vi "FromRepo.vi"(8 "error in":errorcluster, 9 "from repo cluster":T2, 10 "repository in":refnum<class "CEF_Repository.lvclass">, 11 "CEF_configuration":refnum<class "CEF_serializable node.lvclass">) -> (0 "error out":errorcluster, 2 "repository out":refnum<class "CEF_Repository.lvclass">, 3 "node":T1)   [LabVIEW 2023, in "CEF.lvlib" / "CEF_serializable node.lvclass"]
doc: "Grabs information from the Repo and stores it in the nodes.Copyright 2017 National Instruments Corporation\n\nLicensed under the Apache License, Version 2.0 (the \"License\"); you may not use this file except in compliance with the License. You may obtain a copy of the License at http://www.apache.org/licenses/LICENSE-2.0\nUnless required by applicable law or agreed to in writing, software distributed under the License is distributed on an \"AS IS\" BASIS, WITHOUT WARRANTIES OR CONDITIONS OF ANY KIND, either express or implied. See the License for the specific language governing permissions and limitations under the License."
uses:
  CEF_serializable node.lvclass
  Repository/CEF_Repository.lvclass
  Node/FromRepoCluster.ctl
  Node/NodeRef.ctl
  Node/CEF_Node.lvclass
  hierarchy repo/CEF_HierarchyRepo.lvclass
  C:/Working Copy/TSS/Utilities/Configuration Framework/Repository/CEF_Repository.lvclass
  serializable configuration/CEF_serializable configuration.lvclass
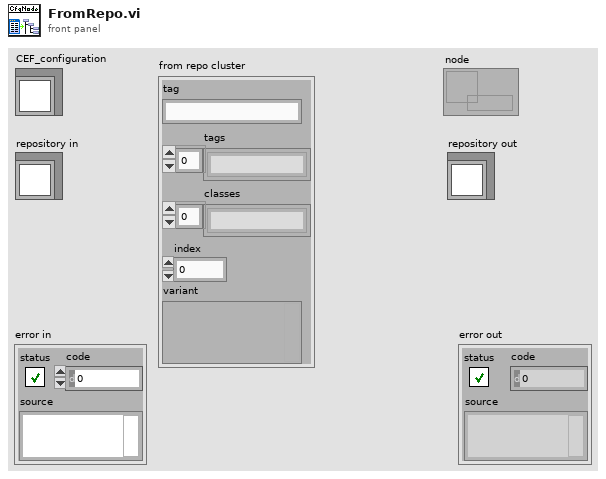
[diagram p1: front panel]
types:
  T1 = typedef "CEF.lvlib/CEF_Node.lvclass/NodeRef.ctl" = refnum<data-value>
  T2 = typedef "CEF.lvlib/CEF_Node.lvclass/FromRepoCluster.ctl" = cluster{"tag":string, "tags":string[], "classes":string[], "index":i32, "variant":variant}
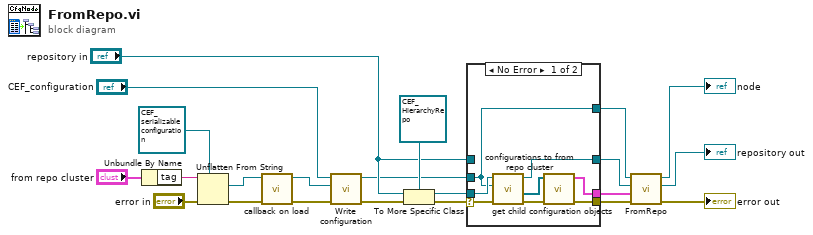
[diagram p0: block diagram]
diagram:
  n1 = Unbundle By Name("from repo cluster") -> ("tag"=w9:string)
  n2 = Unflatten From String(type=refnum<class "CEF_serializable configuration.lvclass"> refnum ("configuration"), binary string=w9, error in (no error)="error in") -> (value=w4:refnum<class "CEF_serializable configuration.lvclass">, error out=w3:errorcluster)  [unwired: 2 in, 1 out]
  n3 = call-dynamic "callback on load.vi"("error in"=w3, "CEF_Configuration in"=w4) -> ("error out"=w2:errorcluster, "CEF_Configuration out"=w1:refnum<class "CEF_serializable configuration.lvclass">)  [unwired: 8 in]
  n4 = call-dynamic "Write configuration.vi"("error in"=w2, "CEF Configuration"=w1, "CEF_serializable node in"="CEF_configuration") -> ("error out"=w6:errorcluster, "CEF_serializable node out"=w5:refnum<class "CEF_serializable node.lvclass">)  [unwired: 7 in]
  n5 = To More Specific Class(target class=refnum<class "CEF_HierarchyRepo.lvclass"> refnum ("CEF_HierarchyRepo.lvclass"), reference="repository in", error in=w6) -> (specific class reference=w20:refnum<class "CEF_HierarchyRepo.lvclass">, error out=w22:errorcluster)
  n6 = case shown="No Error" w22 {
    selector: w22 -> [w28 w32]
    tunnel: "repository in" -> [_ w33]
    tunnel: [w29 w33] -> w17
    tunnel: [w26 w32] -> w19
    tunnel: w5 -> [w23 w31]
    tunnel: [w23 w31] -> w18
    tunnel: w20 -> [w30 _]
    tunnel: [w24 _] -> w12
    frame No Error {
      n7 = call-dynamic "get child configuration objects.vi"("error in"=w28, "serializable node"=w23, "CEF_HierarchyRepo in"=w30) -> ("error out"=w27:errorcluster, "children"=w25:refnum<class "CEF_serializable configuration.lvclass">[], "CEF_HierarchyRepo out"=w29:refnum<class "CEF_HierarchyRepo.lvclass">)  [unwired: 6 in]
      n8 = call "configurations to from repo cluster.vi"("error in"=w27, "configurations"=w25) -> ("error out"=w26:errorcluster, "from repo cluster"=w24:T2)  [unwired: 8 in]
    }
    frame Error {
    }
  }
  n9 = call-parent "FromRepo.vi"("error in"=w19, "from repo cluster"=w12, "repository in"=w17, "CEF_Node in"=w18) -> ("error out"=→"error out":errorcluster, "repository out"=→"repository out":refnum<class "CEF_Repository.lvclass">, "node"=→"node":T1)  [unwired: 5 in]
